vi "set_z_step_size.vi"(8 "error in (no error)":errorcluster, 9 "z-offset":u16, 10 "z-step size / frame":u16, 11 "TrajectoryMH100122AODRAPS in":refnum<class "TrajectoryMH100122AODRAPS.lvclass">) -> (0 "error out":errorcluster, 3 "TrajectoryMH100122AODRAPS out":refnum<class "TrajectoryMH100122AODRAPS.lvclass">)   [LabVIEW 2010, in "TrajectoryMH100122AODRAPS.lvclass"]
uses:
  TrajectoryMH100122AODRAPS.lvclass
  TrajectoryMH100122AODRAPS.lvclass/TrajectoryMH100122AODRAPS.ctl
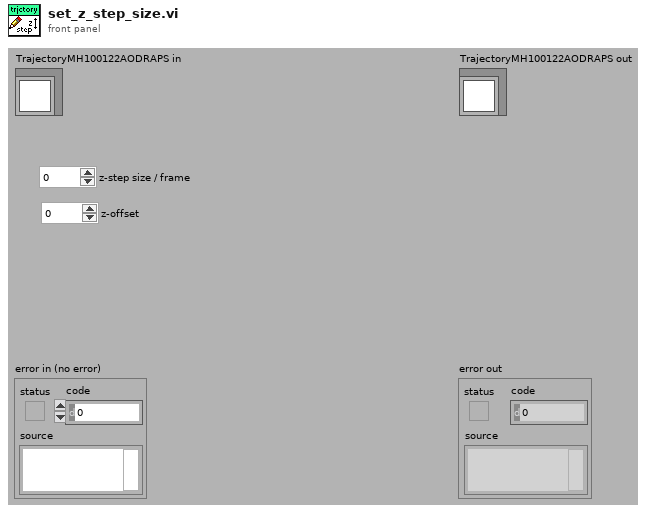
[diagram p1: front panel]
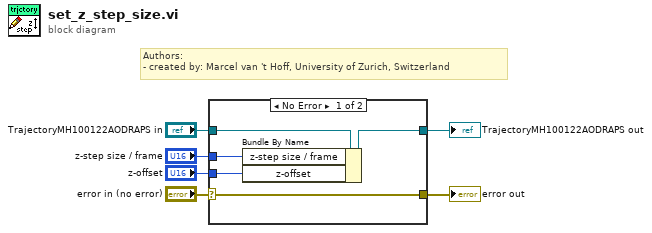
[diagram p0: block diagram]
diagram:
  # "Authors: \n- created by: Marcel van 't Hoff, University of Zurich, Switzerland"
  n1 = case shown="No Error" "error in (no error)" {
    selector: "error in (no error)" -> [w11 w13]
    tunnel: [w11 w13] -> w5
    tunnel: [w8 w12] -> w3
    tunnel: "TrajectoryMH100122AODRAPS in" -> [w9 w12]
    tunnel: "z-step size / frame" -> [w10 _]
    tunnel: "z-offset" -> [w7 _]
    frame No Error {
      n2 = Bundle By Name(cluster=w9, "z-step size / frame"=w10, "z-offset"=w7) -> (w8:refnum<class "TrajectoryMH100122AODRAPS.lvclass">)
    }
    frame Error {
    }
  }
  "error out" <- w5
  "TrajectoryMH100122AODRAPS out" <- w3
